vi "test_fxpAverageSCTL.vi"() -> ()   [LabVIEW 2016]
uses:
  <vilib>/rvi/DesktopExecutionNode/Execution/niFpgaDEN_Execute.vi
  <vilib>/rvi/DesktopExecutionNode/DesktopExecutionNode.xnode
panel:
  out "accumulatorState":fxp<+/-,38,16>[](array[numeric])
  out "Array 6":fxp<+/-,38,17>[][](array[numeric])
  out "inValid":bool[](array[boolean])
  out "Array 5":fxp<+/-,22,1>[](array[numeric])
  out "Array 4":u16[](array[numeric])
  out "Array 3":bool[](array[boolean])
  out "Array 2":fxp<+/-,22,1>[](array[numeric])
  out "average":fxp<+/-,22,1>
  out "Waveform Graph 2":dbl[](graph)
  out "Waveform Graph":dbl[](graph)
  out "Error Out":errorcluster
  out "Array":bool[](array[boolean])
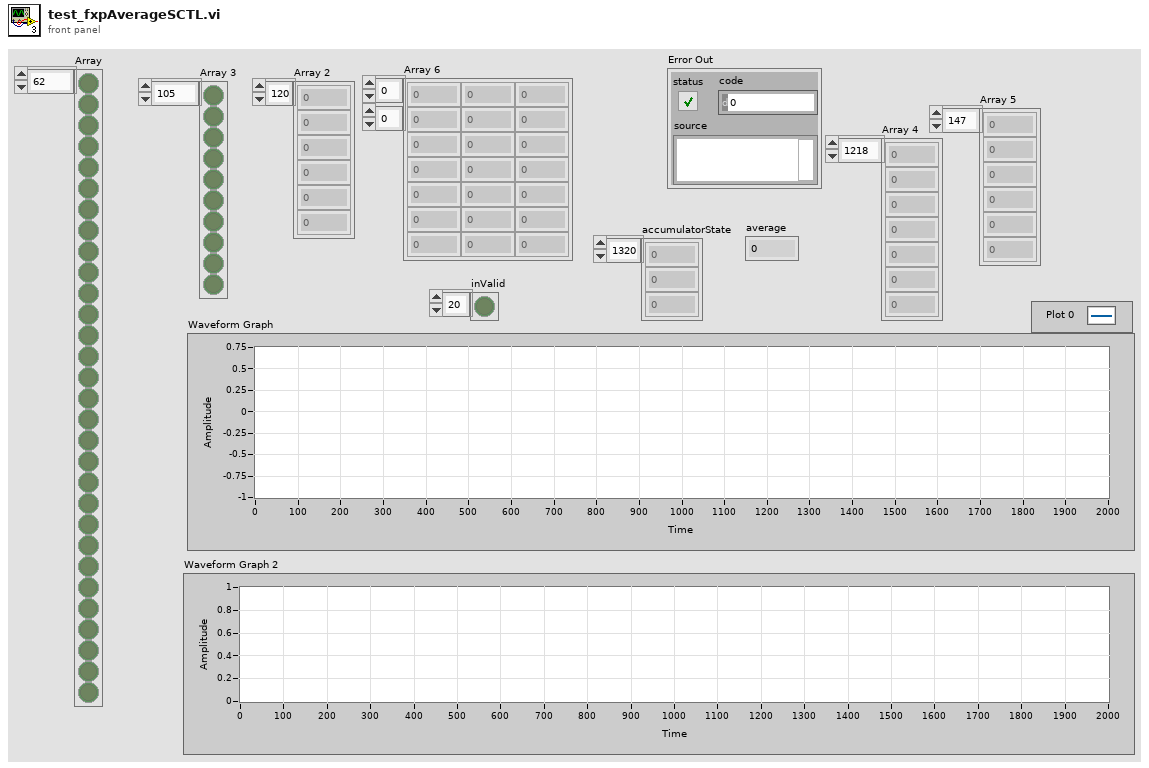
[diagram p1: front panel]
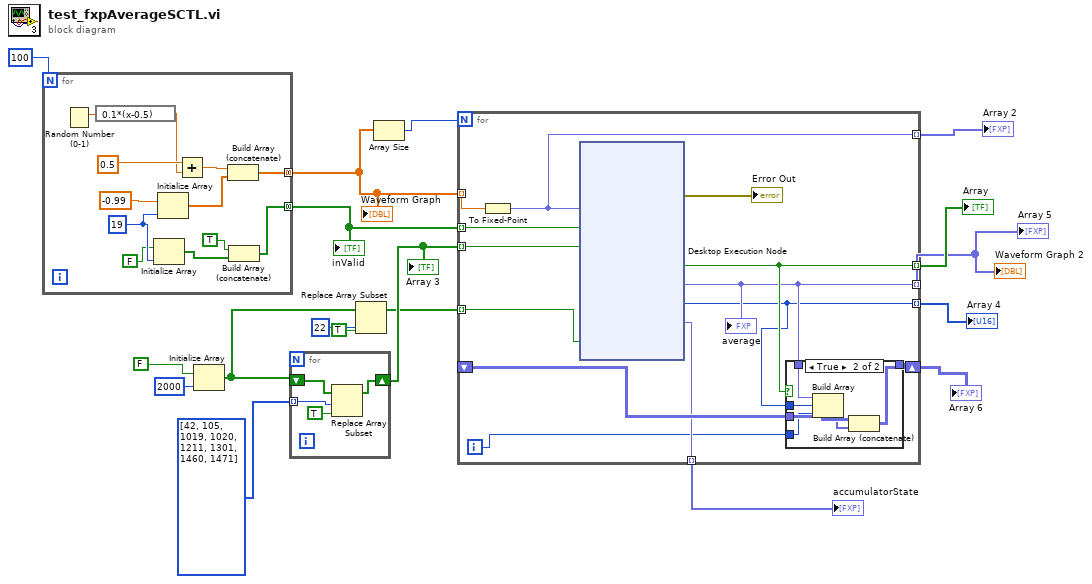
[diagram p0: block diagram]
diagram:
  n1 = for {
    N: 100 -> [_]
    tunnel: [w20] -> w17 mode=concatenating
    tunnel: [w19] -> w11 mode=concatenating
    w24 = 19 ("dimension size")
    n2 = Random Number (0-1)() -> (number: 0 to 1=w29:dbl)
    n3 = expression code="0.1*(x-0.5)"(w29) -> (w28:dbl)
    n4 = Initialize Array(FALSE, w24) -> (w21:bool[])
    n5 = Initialize Array(-0.99, w24) -> (w25:dbl[])
    n6 = Add(x=0.5, y=w28) -> (x+y=w27:dbl)
    n7 = Build Array (concatenate)(w27, w25) -> (w19:dbl[])
    n8 = Build Array (concatenate)(TRUE, w21) -> (w20:bool[])
  }
  "Waveform Graph" <- w11
  "inValid" <- w17
  n9 = Initialize Array(FALSE, 2000 ("dimension size")) -> (w4:bool[])
  n10 = for {
    shift-right: [w33] -> w15
    shift-left: w4 -> [w34]
    tunnel: i32[] [42, 105, 1019, 1020, 1211, 1301, 1460, 1471] -> [w31] mode=indexing
    n11 = Replace Array Subset(array=w34, new element=TRUE ("new element/subarray"), index=w31) -> (w33:bool[])
  }
  "Array 3" <- w15
  n12 = Replace Array Subset(array=w4, new element=TRUE ("new element/subarray"), index=22) -> (w1:bool[])
  n13 = Array Size(array=w11) -> (size(s)=w10:i32)
  n14 = for {
    N: w10 -> [_]
    tunnel: w17 -> [w47] mode=indexing
    tunnel: w11 -> [w46] mode=indexing
    tunnel: w15 -> [w45] mode=indexing
    tunnel: [w42] -> w13 mode=indexing
    tunnel: [w41] -> w12 mode=indexing
    tunnel: [w43] -> w9 mode=indexing
    tunnel: [w40] -> w7 mode=indexing
    shift-right: [w38] -> w6
    shift-left: _ -> [w39]
    tunnel: [w37] -> w5 mode=indexing
    tunnel: w1 -> [w36] mode=indexing
    i -> [w35]
    n15 = To Fixed-Point(number=w46) -> (fixed-point=w43:fxp<+/-,22,1>)  [unwired: 1 in]
    n16 = xnode "Desktop Execution Node"("input"=w43, "inputValid"=w47, "reset"=w45, "clear"=w36) -> ("Error Out"=→"Error Out":errorcluster, "outputValid"=w42:bool, "average"=w41:fxp<+/-,22,1>, "noAvg"=w40:u16, "x+y"=w37:fxp<+/-,38,16>)  [unwired: 1 in]
    "average" <- w41
    n17 = case shown="True" w42 {
      tunnel: w41 -> [_ w54]
      tunnel: w40 -> [_ w53]
      tunnel: w39 -> [w48 w52]
      tunnel: [w48 w50] -> w38
      tunnel: w35 -> [_ w49]
      frame False {
      }
      frame True {
        n18 = Build Array(w54, w53, w49) -> (w51:fxp<+/-,53,32>[])
        n19 = Build Array (concatenate)(w52, w51) -> (w50:fxp<+/-,53,32>[][])
      }
    }
  }
  "Array" <- w13
  "Waveform Graph 2" <- w12
  "Array 2" <- w9
  "Array 4" <- w7
  "Array 5" <- w12
  "Array 6" <- w6
  "accumulatorState" <- w5
